vi "Compare Response.vi"(10 "Actual":refnum<class "CANopen Response Message.lvclass">, 11 "Service Data Object":refnum<class "Service Data Object.lvclass">) -> (2 "Equal?":bool, 3 "Service Data Object out":refnum<class "Service Data Object.lvclass">)   [LabVIEW 2024, in "CANopen Master.lvlib" / "Service Data Object.lvclass"]
uses:
  Service Data Object.lvclass
  Service Data Object.lvclass/Service Data Object.ctl
  SDO Response Compare Strategy/SDO Response Compare Strategy.lvclass
  CANopen Response/CANopen Response Message.lvclass
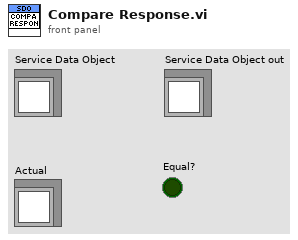
[diagram p1: front panel]
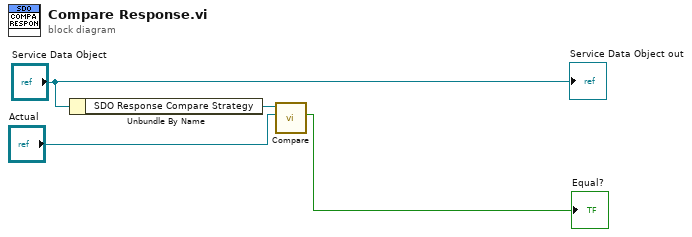
[diagram p0: block diagram]
diagram:
  n1 = Unbundle By Name("Service Data Object") -> ("SDO Response Compare Strategy"=w3:refnum<class "SDO Response Compare Strategy.lvclass">)
  n2 = call-dynamic "Compare.vi"("Actual"="Actual", "SDO Response Compare Strategy in"=w3) -> ("Equal?"=→"Equal?":bool)  [unwired: 7 in, 2 out]
  "Service Data Object out" <- "Service Data Object"
